vi "Read Mean Std.vi"(8 "error in (no error)":errorcluster, 11 "Display Image in":refnum<class "Display Image.lvclass">) -> (0 "error out":errorcluster, 1 "Stddev":dbl, 2 "Mean":dbl, 3 "Display Image out":refnum<class "Display Image.lvclass">)   [LabVIEW 2018, in "Display Image.lvclass"]
doc: "Este VI faz a leitura da média e desvio padrão contidos na classe."
uses:
  Display Image.lvclass
  Display Image.lvclass/Display Image.ctl
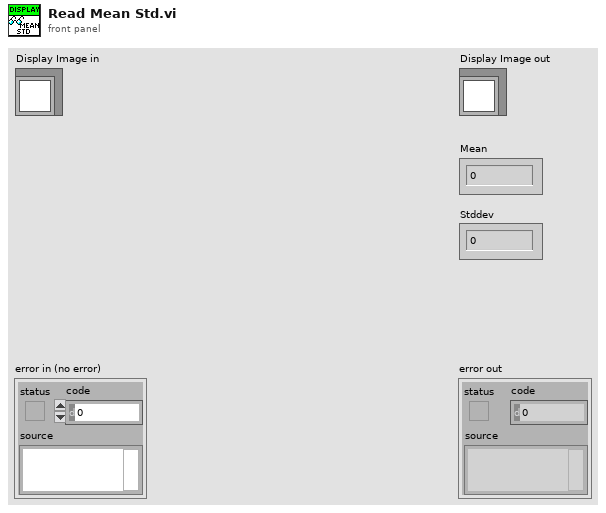
[diagram p1: front panel]
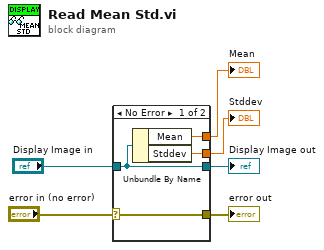
[diagram p0: block diagram]
diagram:
  n1 = case shown="No Error" "error in (no error)" {
    selector: "error in (no error)" -> [w10 w11]
    tunnel: [w10 w11] -> w5
    tunnel: [w9 w12] -> w3
    tunnel: "Display Image in" -> [w9 w12]
    tunnel: [w8 _] -> w2
    tunnel: [w7 _] -> w1
    frame No Error {
      n2 = Unbundle By Name(w9) -> ("Mean"=w8:dbl, "Stddev"=w7:dbl)
    }
    frame Error {
    }
  }
  "error out" <- w5
  "Display Image out" <- w3
  "Mean" <- w2
  "Stddev" <- w1
